vi "getCurrent.vi"(3 "error in (no error)":errorcluster, 4 "Throttle % [0-100]":dbl, 5 "ACS759 in":refnum<class "ACS759.lvclass">) -> (0 "error out":errorcluster, 1 "Current [Amps]":dbl, 2 "ACS759 out":refnum<class "ACS759.lvclass">)   [LabVIEW 2015, in "ACS759.lvclass"]
uses:
  ACS759.lvclass
panel:
  out "Current [Amps] 2":dbl
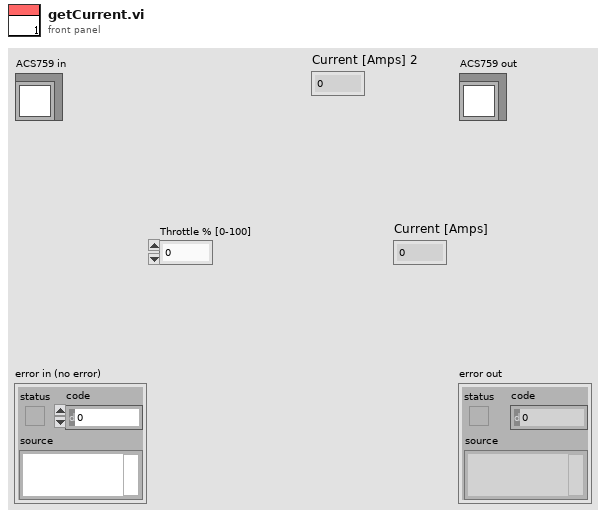
[diagram p1: front panel]
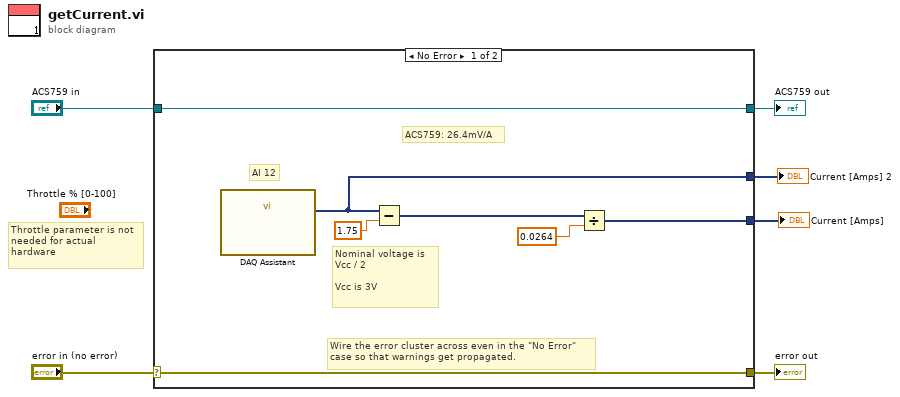
[diagram p0: block diagram]
diagram:
  # "Throttle parameter is not\nneeded for actual \nhardware"
  n1 = case shown="No Error" "error in (no error)" {
    selector: "error in (no error)" -> [w12 w15]
    tunnel: [w12 w15] -> w5
    tunnel: [w13 w14] -> w3
    tunnel: "ACS759 in" -> [w13 w14]
    tunnel: [w10 _] -> w2
    tunnel: [w7 _] -> w1
    frame No Error {
      # "Nominal voltage is \nVcc / 2\n\nVcc is 3V"
      # "ACS759: 26.4mV/A"
      # "AI 12"
      # "Wire the error cluster across even in the \"No Error\"\ncase so that warnings get propagated."
      n2 = call "DAQ Assistant"() -> ("data"=w7:dynamicdata)  [unwired: 17 in, 2 out]
      n3 = Subtract(x=w7, y=1.75) -> (x-y=w8:dynamicdata)
      n4 = Divide(x=w8, y=0.0264) -> (x/y=w10:dynamicdata)
    }
    frame Error {
    }
  }
  "error out" <- w5
  "ACS759 out" <- w3
  "Current [Amps]" <- w2
  "Current [Amps] 2" <- w1
